vi "PathPlanner_PathFinder_DoMajor.vi"   [LabVIEW 2019]
uses:
  <vilib>/Utility/miscctls.llb/LVMapReplaceAction.ctl
  PathPlannerLib24/VI/PathPlanner_PathFinder_TopKey.vi
  PathPlannerLib24/VI/PathPlanner_PathFinder_ComparePair.vi
  PathPlannerLib24/VI/PathPlanner_GridPosition_HashCode.vi
  PathPlannerLib24/VI/PathPlanner_PathFinder_UpdateState.vi
  PathPlannerLib24/VI/PathPlanner_PathFinder_GetOpenNeighbors.vi
  PathPlannerLib24/VI/PathPlanner_GridPosition_Equals.vi
  PathPlannerLib24/VI/PathPlanner_PathFinder_GridPosToTranslation2d.vi
  <vilib>/Rock Robotics/WPI/ThirdParty/JAS_Junk/TrajLib/Translation2d_GetDistance.vi
  PathPlannerLib24/VI/PathPlanner_PathFinder_Constants.vi
  <vilib>/Rock Robotics/WPI/ThirdParty/JAS_Junk/TrajLib/Translation2d_Create_DistAng.vi
  <vilib>/Rock Robotics/WPI/ThirdParty/JAS_Junk/TrajLib/Translation2d_Minus.vi
  <vilib>/Rock Robotics/WPI/ThirdParty/JAS_Junk/TrajLib/Translation2d_GetAngle.vi
  <vilib>/Rock Robotics/WPI/ThirdParty/JAS_Junk/TrajLib/Translation2d_Plus.vi
  PathPlannerLib24/VI/PathPlanner_PathFinder_ExtractPathSub1ALT.vi
  PathPlannerLib24/VI/PathPlanner_PathFinder_IsWalkable.vi
  PathPlannerLib24/VI/PathPlanner_PathFinder_Heuristic.vi
  PathPlannerLib24/VI/PathPlanner_GridPosition_New.vi
  PathPlannerLib24/VI/PathPlanner_GridPosition_Get.vi
  PathPlannerLib24/VI/PathPlanner_PathFinder_Cost.vi
  <vilib>/Rock Robotics/WPI/ThirdParty/JAS_Junk/TrajLib/Translation2d_Create.vi
  <vilib>/Rock Robotics/WPI/ThirdParty/JAS_Junk/TrajLib/Util_CalcDist.vi
  <vilib>/Rock Robotics/WPI/ThirdParty/JAS_Junk/TrajLib/Rotation2d_GetAngleCosSin.vi
  <vilib>/Rock Robotics/WPI/ThirdParty/JAS_Junk/TrajLib/Translation2d_GetXY.vi
  <vilib>/Rock Robotics/WPI/ThirdParty/JAS_Junk/TrajLib/Rotation2d_CreateXY.vi
  PathPlannerLib24/VI/PathPlanner_PathFinder_IsCollision.vi
  PathPlannerLib24/VI/PathPlanner_GridPosition_Print.vi
  <vilib>/robotics/Navigation/shared/MapNode/AbstractDstarNode/NI_Robotics_AbstractDstarNode.lvclass
  C:/Program Files/National Instruments/LabVIEW 2019/vi.lib/robotics/Navigation/shared/MapNode/AbstractAstarNode/NI_Robotics_AbstractAstarNode.lvclass
  PathPlannerLib24/VI/PathPlanner_PathFinder_Globals.vi
  <vilib>/robotics/Navigation/shared/WorldMap/OccupancyGridWorldMap/Get Cells in Path.vi
  PathPlannerLib24/VI/PathPlanner_PathFinder_ApplyControlSmooth.vi
  PathPlannerLib24/VI/PathPlanner_PathFinder_ApplyAnchorSmooth.vi
  PathPlannerLib24/PathPlanner24.lvlib
types:
  T1 = typedef "LVMapReplaceAction.ctl" = enum32{"Modify Entry only if found", "Add or Modify Entry", "Delete Entry"}
  T2 = typedef "PathPlanner24.lvlib/PathPlannerFinderDoublePair.ctl" = cluster{"A":dbl, "B":dbl}
  T3 = typedef "PathPlanner24.lvlib/PathPlannerFinderGridPosition.ctl" = cluster{"X":i32, "Y":i32}
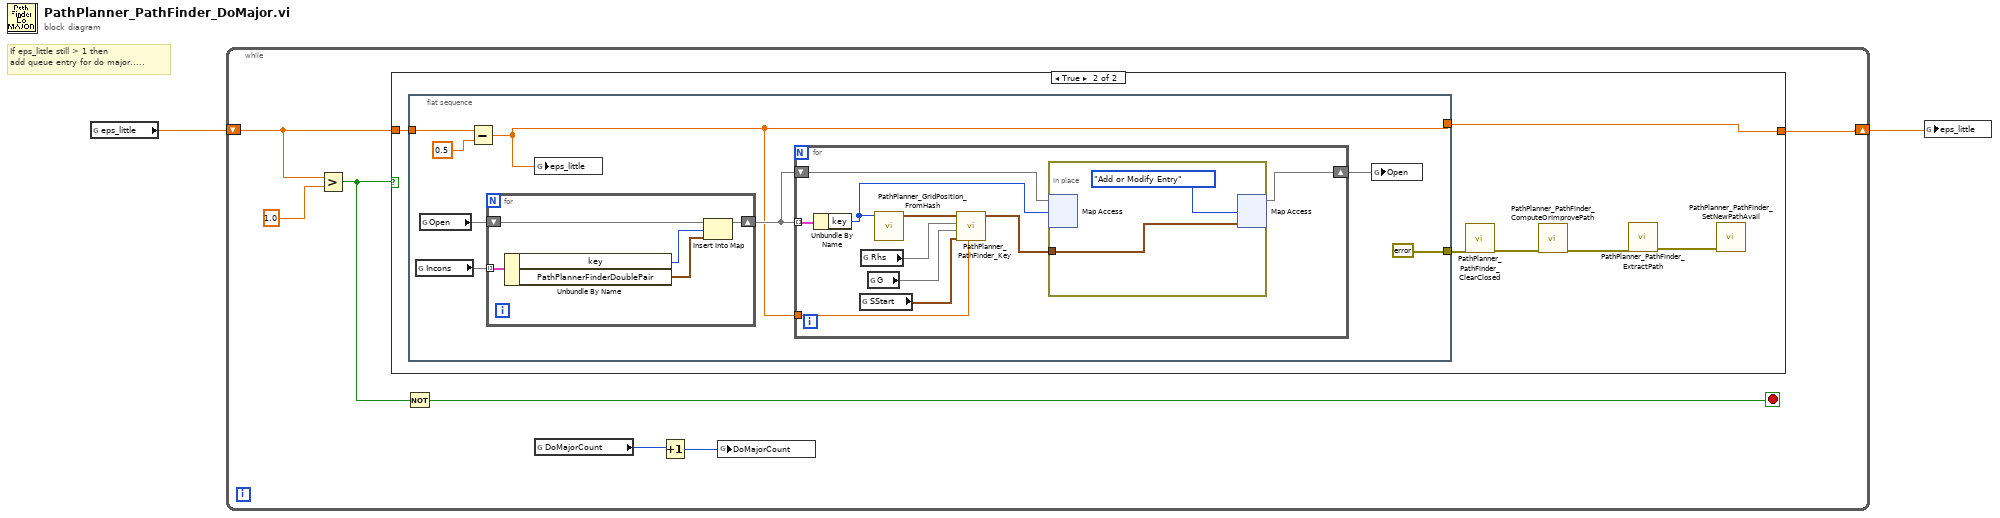
[diagram p0: block diagram]
diagram:
  # "If eps_little still > 1 then\nadd queue entry for do major....."
  n1 = global read "PathPlanner_PathFinder_Globals.vi" "eps_little"() -> (w2:dbl)
  n2 = while {
    shift-right: [w7] -> w1
    shift-left: w2 -> [w8]
    stop <- w5 stop-if-true
    n3 = Greater?(x=w8, y=1.0) -> (0:w6:bool)
    n4 = case shown="True" w6 {
      tunnel: w8 -> [w10 w16]
      tunnel: [w10 w12] -> w7
      frame False {
      }
      frame True {
        n5 = flat-sequence {
          tunnel: w16 -> [w24]
          tunnel: [w17] -> w12
          tunnel: [errorcluster {"status"=FALSE, "code"=0, "source"=""} ("error in (no error)")] -> w11
          frame #0 {
            n6 = global read "PathPlanner_PathFinder_Globals.vi" "Incons"() -> (w22:map{i32, T2})
            n7 = global read "PathPlanner_PathFinder_Globals.vi" "Open"() -> (w21:map{i32, T2})
            n8 = Subtract(x=w24, y=0.5) -> (x-y=w17:dbl)
            n9 = for {
              tunnel: w22 -> [w40] mode=indexing
              shift-right: [w39] -> w20
              shift-left: w21 -> [w41]
              n10 = Unbundle By Name(w40) -> ("key"=w38:i32, "PathPlannerFinderDoublePair"=w37:T2)
              n11 = Insert Into Map(map in=w41, key=w38, value=w37) -> (map out=w39:map{i32, T2})  [unwired: 2 out]
            }
            n12 = global write "PathPlanner_PathFinder_Globals.vi" "eps_little"(w17) -> ()
            n13 = for {
              tunnel: w20 -> [w33] mode=indexing
              shift-right: [w27] -> w19
              shift-left: w20 -> [w25]
              tunnel: w17 -> [w26]
              n14 = Unbundle By Name(w33) -> ("key"=w28:i32)
              n15 = global read "PathPlanner_PathFinder_Globals.vi" "SStart"() -> (w30:T3)
              n16 = global read "PathPlanner_PathFinder_Globals.vi" "Rhs"() -> (w32:map{i32, dbl})
              n17 = global read "PathPlanner_PathFinder_Globals.vi" "G"() -> (w31:map{i32, dbl})
              n18 = call "PathPlanner_GridPosition_FromHash.vi"("Hash"=w28) -> ("GridPosition"=w34:T3)  [unwired: 10 in]
              n19 = call "PathPlanner_PathFinder_Key.vi"("eps_little"=w26, "Sstart"=w30, "G"=w31, "RHS"=w32, "S"=w34) -> ("DoublePair"=w29:T2)  [unwired: 6 in]
              n20 = in-place {
                in-place-border: w29 -> [w35]
                n21 = in-place-map #1(w25, w28) -> ()  [unwired: 1 in, 2 out]
                n22 = in-place-map #1(w35, LVMapReplaceAction."Add or Modify Entry" ("action")) -> (w27:map{i32, T2})  [unwired: 2 out]
              }
            }
            n23 = global write "PathPlanner_PathFinder_Globals.vi" "Open"(w19) -> ()
          }
        }
        n24 = call "PathPlanner_PathFinder_ClearClosed.vi"("error in (no error)"=w11) -> ("error out"=w13:errorcluster)  [unwired: 10 in]
        n25 = call "PathPlanner_PathFinder_ComputeOrImprovePath.vi"("error in (no error)"=w13) -> ("error out"=w14:errorcluster)  [unwired: 10 in]
        n26 = call "PathPlanner_PathFinder_ExtractPath.vi"("error in (no error)"=w14) -> ("error out"=w15:errorcluster)  [unwired: 10 in]
        n27 = call "PathPlanner_PathFinder_SetNewPathAvail.vi"("error in (no error)"=w15) -> ()  [unwired: 10 in, 1 out]
      }
    }
    n28 = Not(x=w6) -> (.not. x?=w5:bool)
    n29 = global read "PathPlanner_PathFinder_Globals.vi" "DoMajorCount"() -> (w4:i64)
    n30 = Increment(x=w4) -> (x+1=w3:i64)
    n31 = global write "PathPlanner_PathFinder_Globals.vi" "DoMajorCount"(w3) -> ()
  }
  n32 = global write "PathPlanner_PathFinder_Globals.vi" "eps_little"(w1) -> ()
